vi "Convert Number to String.vi"(1 "Numeric":i32) -> (0 "String":string)   [LabVIEW 2019, in "Instrument UI.PPMS.lvclass"]
uses:
  Instrument UI.PPMS.lvclass
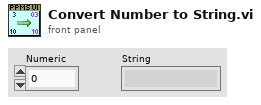
[diagram p1: front panel]
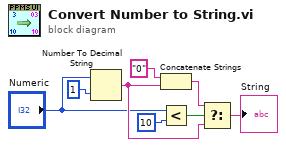
[diagram p0: block diagram]
diagram:
  n1 = Number To Decimal String(number="Numeric", width (-)=i16 1) -> (decimal integer string=w6:string)
  n2 = Concatenate Strings("0" ("string"), w6) -> (w8:string)
  n3 = Less?(x="Numeric", y=10) -> (x < y?=w4:bool)
  n4 = Select(t=w8, s=w4, f=w6) -> (s? t:f=→"String":string)
